vi "Set Msg Received Event.vi"(8 "error in":errorcluster, 10 "Msg Received Event":refnum<user-event>, 11 "Logger in":refnum<class "Logger.lvclass">) -> (0 "error out":errorcluster, 3 "Logger out":refnum<class "Logger.lvclass">)   [LabVIEW 2020, in "CANopen Logging.lvlib" / "Logger.lvclass"]
uses:
  Logger.lvclass
  Logger.lvclass/Logger.ctl
  HAL/Source/Interfaces/IMessage/IMessage.lvclass
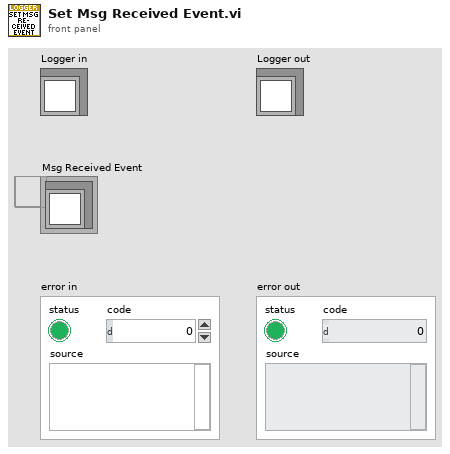
[diagram p1: front panel]
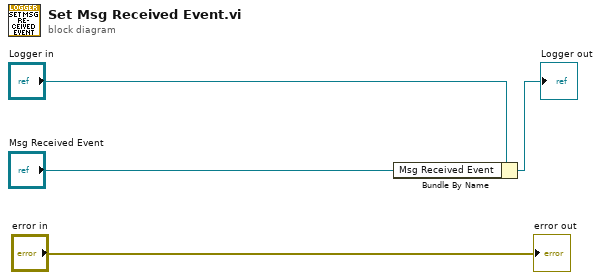
[diagram p0: block diagram]
diagram:
  n1 = Bundle By Name(cluster="Logger in", "Msg Received Event"="Msg Received Event") -> (→"Logger out":refnum<class "Logger.lvclass">)
  "error out" <- "error in"
